vi "IIR Filter (DBL).vi"(2 "init/cont (init:F)":bool, 3 "Forward Coefficients":dbl[](array[numeric]), 4 "Reverse Coefficients":dbl[](array[numeric]), 5 "X":dbl[](array[numeric])) -> (0 "error":i32, 1 "Filtered X":dbl[](array[numeric]))   [LabVIEW 2020, in "NI_AALBase.lvlib"]
doc: "Filters the input sequence <B>X</B> using the direct form IIR filter specified by <B>Reverse Coefficients</B> and <B>Forward Coefficients</B>. Wire data to the <B>X</B> input to determine the polymorphic instance to use or manually select the instance."
uses:
  NI_AALBase.lvlib
  <resource>/lvanlys.dll
panel:
  # "IIR Filter"
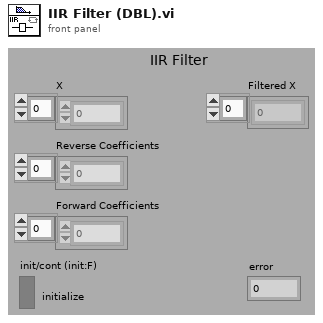
[diagram p1: front panel]
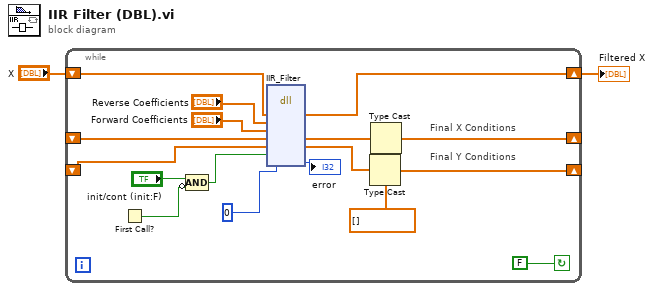
[diagram p0: block diagram]
diagram:
  n1 = while {
    shift-left: _ -> [w10]
    shift-right: [w18] -> _
    shift-left: _ -> [w12]
    shift-right: [w19] -> _
    shift-right: [w3] -> w1
    shift-left: "X" -> [w4]
    stop <- FALSE continue-if-true
    w17 = dbl[] [] ("type for the shift register")
    # "Final Y Conditions"
    # "Final X Conditions"
    n2 = First Call?() -> (First Call?: T/F=w6:bool)
    n3 = Compound Arithmetic op=AND("init/cont (init:F)", invert w6) -> (w5:bool)
    n4 = dll-call lib="C:/Program Files (x86)/National Instruments/LabVIEW 2020/resource/lvanlys.*" fn="IIR_Filter"("X"=w4, "Reverse Coefficients"="Reverse Coefficients", "Forward Coefficients"="Forward Coefficients", "type for the shift register"=w12, "type for the shift register"=w10, w5, 0) -> ("X"=w3:dbl[], "type for the shift register"=w11:dbl[], "type for the shift register"=w9:dbl[], →"error":i32)  [unwired: 7 in, 2 out]
    n5 = Type Cast(type=w17, x=w9) -> (*(type *) &x=w18:dbl[])
    n6 = Type Cast(type=w17, x=w11) -> (*(type *) &x=w19:dbl[])
  }
  "Filtered X" <- w1
